vi "GAME_generatePuzzleAndSolution.vi"(8 "error in (no error)":errorcluster) -> (0 "error out":errorcluster, 2 "Solution":string="INTERSTELLAR", 3 "Puzzle":string)   [LabVIEW 2020]
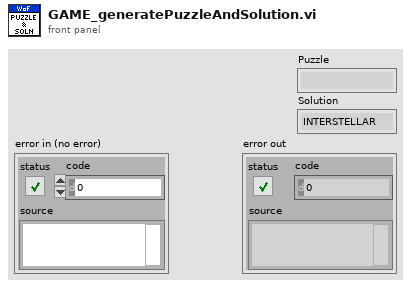
[diagram p1: front panel]
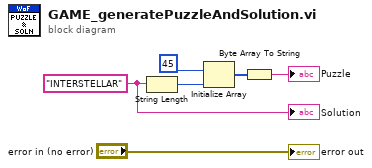
[diagram p0: block diagram]
diagram:
  w5 = "INTERSTELLAR"
  n1 = String Length(string=w5) -> (length=w6:i32)
  n2 = Initialize Array(u8 45, w6) -> (w2:u8[])
  n3 = Byte Array To String(unsigned byte array=w2) -> (string=→"Puzzle":string)
  "Solution" <- w5
  "error out" <- "error in (no error)"
